vi "GetCloseEventRef.vi"(8 "error in (no error)":errorcluster, 11 "VIActivation in":refnum<class "VIActivation.lvclass">) -> (0 "error out":errorcluster, 2 "CloseEventRef out":refnum<user-event>, 3 "VIActivation out":refnum<class "VIActivation.lvclass">)   [LabVIEW 2021, in "VIActivation.lvlib" / "VIActivation.lvclass"]
uses:
  VIActivation.lvclass
  VIActivation.lvclass/VIActivation.ctl
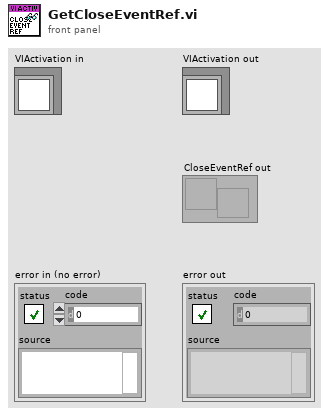
[diagram p1: front panel]
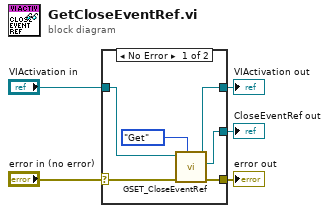
[diagram p0: block diagram]
diagram:
  n1 = case shown="No Error" "error in (no error)" {
    selector: "error in (no error)" -> [w11 w13]
    tunnel: [w10 w13] -> w4
    tunnel: [w9 w12] -> w2
    tunnel: "VIActivation in" -> [w8 w12]
    tunnel: [w6 _] -> w1
    frame No Error {
      n2 = call "GSET_CloseEventRef.vi"("Action"=enum16{"Get", "Set"}."Get", "error in (no error)"=w11, "Menu in"=w8) -> ("error out"=w10:errorcluster, "CloseEventRef out"=w6:refnum<user-event>, "Menu out"=w9:refnum<class "VIActivation.lvclass">)  [unwired: 6 in]
    }
    frame Error {
    }
  }
  "error out" <- w4
  "VIActivation out" <- w2
  "CloseEventRef out" <- w1
